vi "Producer Loop Guard Clause.vi"(8 "error in (no error)":errorcluster, 11 "queue in":refnum<queue>) -> (0 "error out":errorcluster, 3 "queue out":refnum<queue>)   [LabVIEW 2020, in "MacroAssert.lvlib" / "FaKI State Machine.lvlib"]
doc: "Handles errors for the Producer Loop. If <B>error in</B> does not contain an error, this VI is a no-op. If an error is present, the state \"Error Handler >> Producer\" will be enqueued, and the data of that state will be the error cluster itself."
uses:
  FaKI State Machine.lvlib
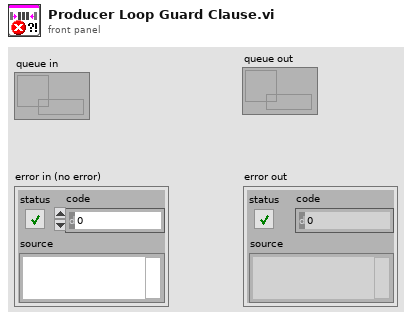
[diagram p1: front panel]
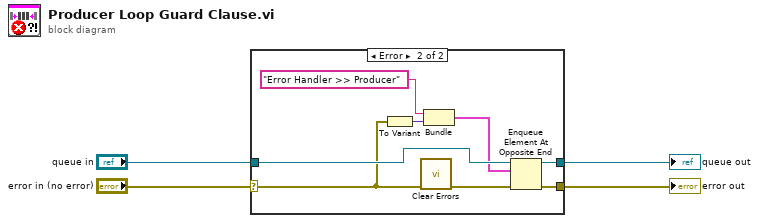
[diagram p0: block diagram]
diagram:
  n1 = case shown="Error" "error in (no error)" {
    selector: "error in (no error)" -> [w6 w10]
    tunnel: [w6 w12] -> w3
    tunnel: "queue in" -> [w5 w11]
    tunnel: [w5 w14] -> w1
    frame No Error {
    }
    frame Error {
      n2 = To Variant(anything=w10) -> (Variant=w8:variant)
      n3 = call <vilib>:"Clear Errors.vi"("error in (no error)"=w10) -> ("error out"=w13:errorcluster)  [unwired: 5 in, 1 out]
      n4 = Bundle("Error Handler >> Producer", "Variant"=w8) -> (w7:cluster{string, "Variant":variant})  [unwired: 1 in]
      n5 = Enqueue Element At Opposite End(queue=w11, element=w7, error in (no error)=w13) -> (queue out=w14:refnum<queue>, error out=w12:errorcluster)  [unwired: 1 in, 1 out]
    }
  }
  "error out" <- w3
  "queue out" <- w1
